vi "TEG P116x1_Write_Auto.vi"(8 "error in (no error)":errorcluster, 9 "NewRT":dbl, 10 "NewSP":dbl, 11 "Comunicaciones":T1={"EUROTHERM"="ASRL6::INSTR", "eur"=FALSE, "ESP32"="ASRL6::INSTR", "esp"=FALSE}) -> (0 "error out":errorcluster, 1 "NewRT":dbl, 2 "NewSP":dbl)   [LabVIEW 2017]
uses:
  cTEG COMMS.ctl
  Eurotherm_New_Module.ctl
  TEG TEST 2022 GLOBALES.vi
panel:
  out "PV":dbl
  out "WorKSP":dbl
  out "TargetSP":dbl
  in  "Cancel":bool
  in  "Write":bool
  # "Programando controlador P116"
  # "C"
  # "C/min"
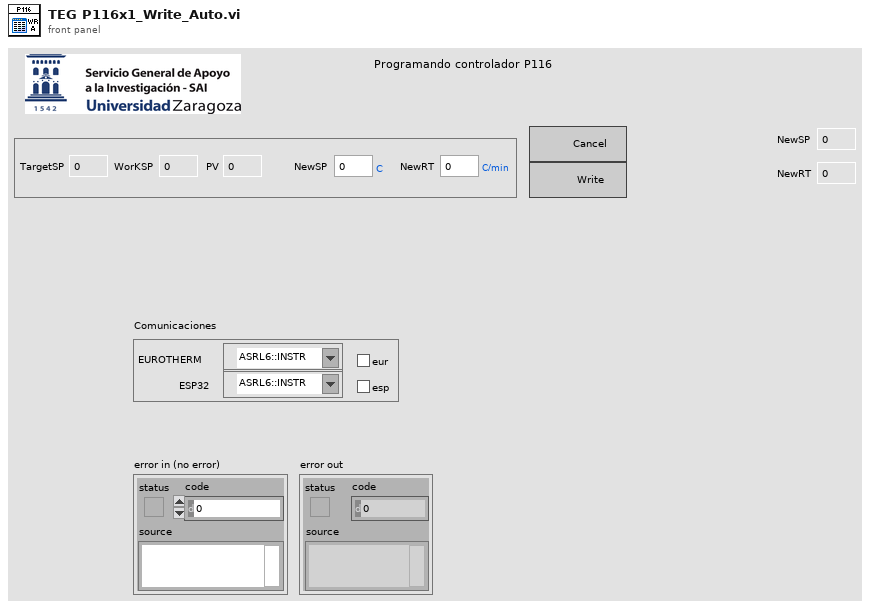
[diagram p1: front panel]
types:
  T1 = typedef "cTEG COMMS.ctl" = cluster{"EUROTHERM":refnum<visa-resource-name>, "eur":bool, "ESP32":refnum<visa-resource-name>, "esp":bool}
  T2 = typedef "TEG P116x1.ctl" = cluster{"TargetSP":dbl, "WorkingSP":dbl, "Temperatura":dbl, "RateSP":dbl, "Potencia":dbl}
  T3 = typedef "Eurotherm_New_Module.ctl" = enum16{"Initialize", "Write SP", "Read SP+PV", "Write Rate", "Set P", "Set I", "Set D", "Shutdown"}
  T4 = enum16{"Add 1", "Add 2", "Add 10", "Add 11", "Add 12", "Add 13"}
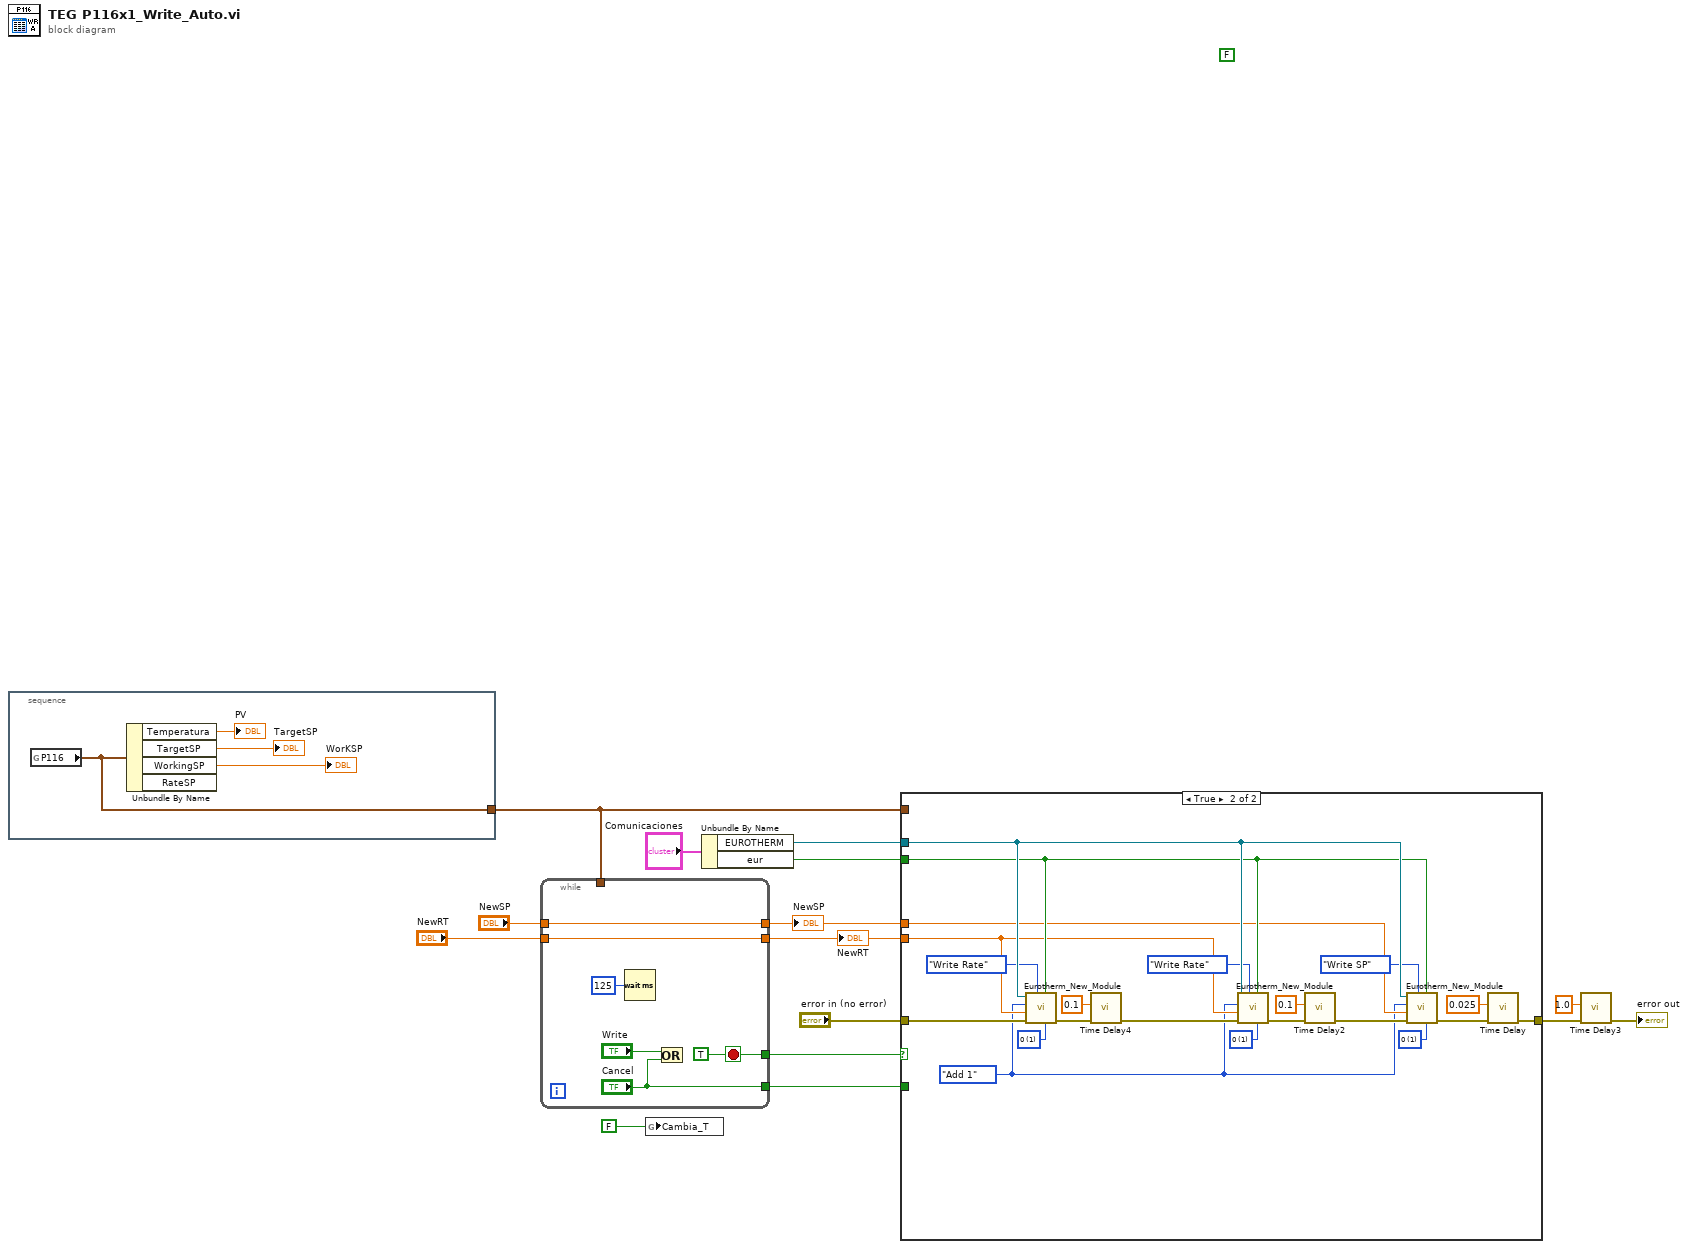
[diagram p0: block diagram]
diagram:
  (unwired) FALSE
  n1 = stacked-sequence {
    tunnel: [w16] -> w10
    frame #0 {
      n2 = global read "TEG TEST 2022 GLOBALES.vi" "P116"() -> (w16:T2)
      n3 = Unbundle By Name(w16) -> ("Temperatura"=→"PV":dbl, "TargetSP"=→"TargetSP":dbl, "WorkingSP"=→"WorKSP":dbl)  [unwired: 1 out]
    }
  }
  n4 = while {
    tunnel: ["Cancel"] -> w14
    tunnel: [w21] -> w2
    tunnel: [w22] -> w1
    tunnel: w10 -> [_]
    tunnel: "NewRT" -> [w22]
    tunnel: "NewSP" -> [w21]
    tunnel: [w20] -> w3
    stop <- w20 stop-if-true
    w20 = TRUE
    n5 = Wait (ms)(milliseconds to wait=u32 125) -> ()  [unwired: 1 out]
    n6 = Or(x="Write", y="Cancel") -> ()  [unwired: 1 out]
  }
  "NewSP" <- w2
  "NewRT" <- w1
  n7 = global write "TEG TEST 2022 GLOBALES.vi" "Cambia_T"(FALSE ("ChangeT")) -> ()
  n8 = Unbundle By Name("Comunicaciones") -> ("EUROTHERM"=w11:refnum<visa-resource-name>, "eur"=w15:bool)
  n9 = case shown="True" w3 {
    tunnel: w15 -> [_ w46]
    tunnel: w14 -> [_ _]
    tunnel: "error in (no error)" -> [w26 w45]
    tunnel: w2 -> [_ w43]
    tunnel: w1 -> [_ w44]
    tunnel: w11 -> [_ w47]
    tunnel: w10 -> [_ _]
    tunnel: [w26 w42] -> w7
    frame False {
    }
    frame True {
      w27 = T4."Add 1" ("Address")
      w28 = u16 1 items=["0"=1, "1"=10, "2"=100] ("Decimales")
      w37 = u16 1 items=["0"=1, "1"=10, "2"=100] ("Decimales")
      w36 = u16 1 items=["0"=1, "1"=10, "2"=100] ("Decimales")
      n10 = call "Eurotherm_New_Module.vi"("Decimales"=w37, "Eurotherm (T:Enable)"=w46, "Command"=Eurotherm_New_Module."Write Rate", "error in (no error)"=w45, "Value"=w44, "Address"=w27, "VISA resource name"=w47) -> ("error out"=w30:errorcluster)  [unwired: 3 in, 1 out]
      n11 = call "Time Delay4"("error in (no error)"=w30, "Delay Time (s)"=0.1) -> ("error out"=w31:errorcluster)  [unwired: 9 in]
      n12 = call "Eurotherm_New_Module.vi"("Decimales"=w28, "Eurotherm (T:Enable)"=w46, "Command"=Eurotherm_New_Module."Write Rate", "error in (no error)"=w31, "Value"=w44, "Address"=w27, "VISA resource name"=w47) -> ("error out"=w29:errorcluster)  [unwired: 3 in, 1 out]
      n13 = call "Time Delay2"("error in (no error)"=w29, "Delay Time (s)"=0.1) -> ("error out"=w34:errorcluster)  [unwired: 9 in]
      n14 = call "Eurotherm_New_Module.vi"("Decimales"=w36, "Eurotherm (T:Enable)"=w46, "Command"=Eurotherm_New_Module."Write SP", "error in (no error)"=w34, "Value"=w43, "Address"=w27, "VISA resource name"=w47) -> ("error out"=w38:errorcluster)  [unwired: 3 in, 1 out]
      n15 = call "Time Delay"("error in (no error)"=w38, "Delay Time (s)"=0.025) -> ("error out"=w42:errorcluster)  [unwired: 9 in]
    }
  }
  n16 = call "Time Delay3"("error in (no error)"=w7, "Delay Time (s)"=1.0) -> ("error out"=→"error out":errorcluster)  [unwired: 9 in]
